vi "StellarNet Init, Read, Close.vi"(0 "Integration Time (ms)":i32=100 caption="Inter scan delay ms", 1 "Use Config\nFile Params (T)":bool, 5 "Number of Scans to Average":i32=1 min=1 max=10000 step=1, 7 "Digitizer Clock Rate Setting":i32=3 min=1 max=3, 9 "Optical Smoothing Level":i32=1 min=0 max=4 step=1, 11 "error in (no error)":errorcluster, 12 "Spectral Channel":i32=1 min=0 max=1 step=1, 14 "Temp  Compensation":bool) -> (4 "Spectrum":cluster{"Wavelengths":dbl[], "buffer out":sgl[]}(graph), 6 "output param":i32, 10 "Critical Error":bool, 15 "error out":errorcluster)   [LabVIEW 2023]
panel:
  # "Use Panel\nParams"
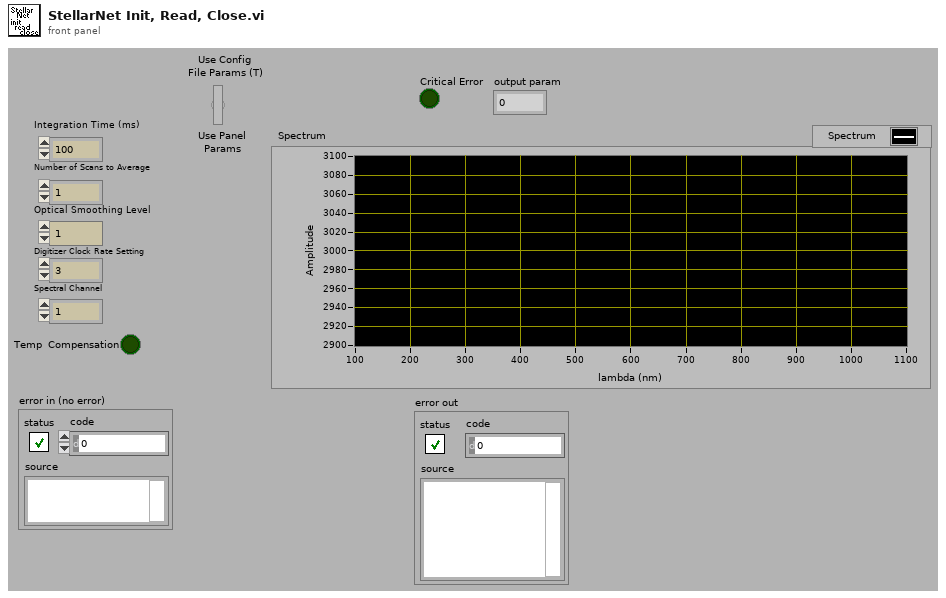
[diagram p1: front panel]
types:
  T1 = cluster{"Coefficients":ext[], "Wavelengths":dbl[]}[]
  T2 = cluster{"Integration Time (ms)":i32, "Number of Scans to Average":i32, "Optical Smoothing Level":i32, "Digitizer Clock Rate Setting":i32, "Temp  Compensation ":bool}[]
  T3 = cluster{"Coefficients":ext[], "Wavelengths":dbl[]}
  T4 = cluster{"Integration Time (ms)":i32, "Number of Scans to Average":i32, "Optical Smoothing Level":i32, "Digitizer Clock Rate Setting":i32, "Temp  Compensation ":bool}
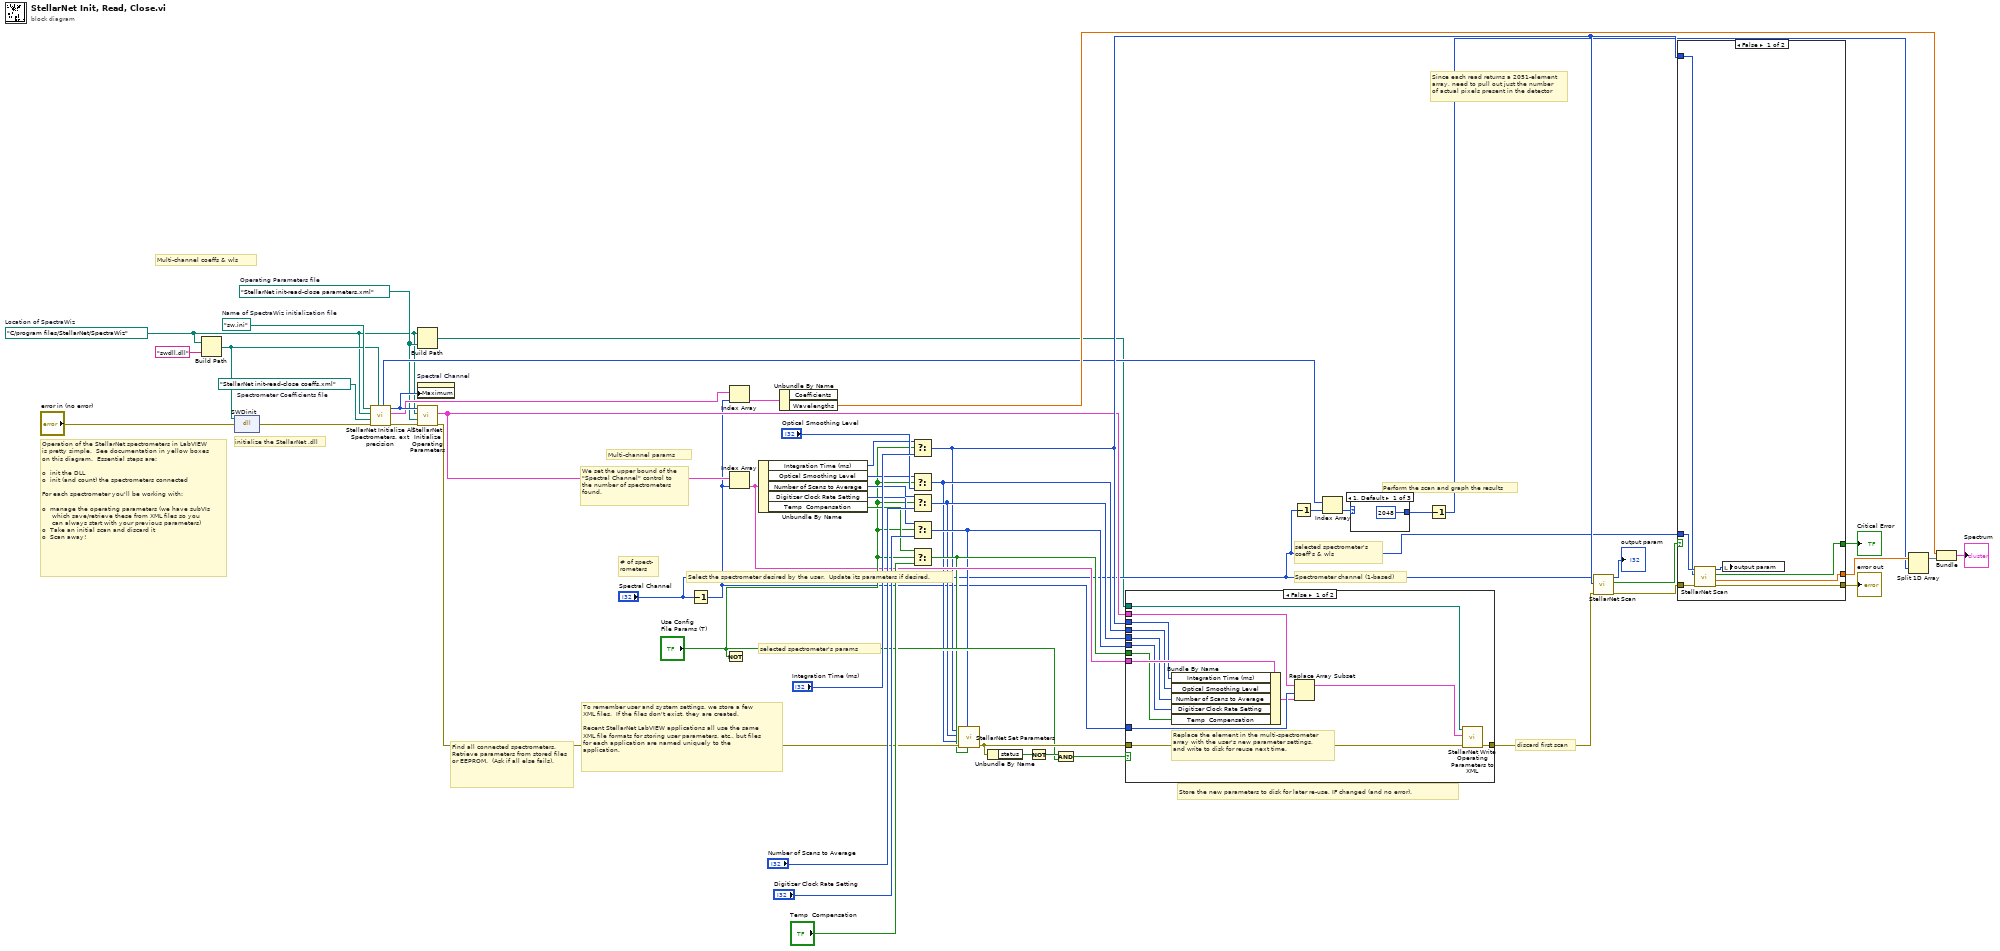
[diagram p0: block diagram]
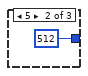
[diagram p2: hidden frame]
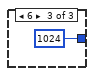
[diagram p3: hidden frame]
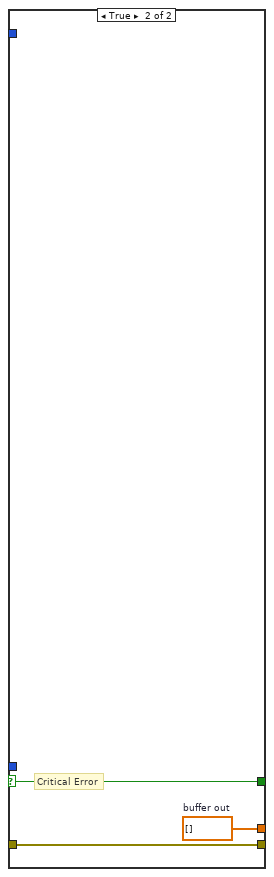
[diagram p5: hidden frame]
diagram:
  w1 = path "C:/program files/StellarNet/SpectraWiz"  # Location of SpectraWiz
  w40 = path "sw.ini"  # Name of SpectraWiz initialization file
  w2 = path "StellarNet init-read-close parameters.xml"  # Operating Parameters file
  w41 = path "StellarNet init-read-close coeffs.xml"  # Spectrometer Coefficients file
  # "Operation of the StellarNet spectrometers in LabVIEW\nis pretty simple.  See documentation in yellow boxes\non this diagram.  Essential steps are:\n\no  init the DLL\no  init (and count) the spectrometers connected\n\nFor each spectrometer you'll be working with:\n\no  manage the operating parameters (we have subVIs\n     which save/retrieve these from XML files so you\n     can always start with your previous parameters)\no  Take an initial scan and discard it\no  Scan away!"
  # "initialize the StellarNet .dll"
  # "Since each read returns a 2051-element\narray, need to pull out just the number\nof actual pixels present in the detector"
  # "Spectrometer channel (1-based)"
  # "Perform the scan and graph the results"
  # "We set the upper bound of the\n\"Spectral Channel\" control to \nthe number of spectrometers \nfound."
  # "To remember user and system settings, we store a few \nXML files.  If the files don't exist, they are created.\n\nRecent StellarNet LabVIEW applications all use the same\nXML file formats for storing user parameters, etc., but files\nfor each application are named uniquely to the \napplication."
  # "Store the new parameters to disk for later re-use, IF changed (and no error)."
  # "Select the spectrometer desired by the user.  Update its parameters if desired."
  # "Find all connected spectrometers.  Retrieve parameters from stored files or EEPROM.  (Ask if all else fails)."
  # "selected spectrometer's\ncoeff's & wls"
  # "Multi-channel coeffs & wls"
  # "selected spectrometer's params"
  # "# of spect-\nrometers"
  # "Multi-channel params"
  # "discard first scan"
  n1 = Build Path(base path=w1, name or relative path="swdll.dll") -> (appended path=w4:path)
  n2 = dll-call lib="C:/Program Files/StellarNet/SpectraWiz/swdll.dll" fn="SWDinit" label="init"(path in=w4, error in="error in (no error)") -> (error out=w6:errorcluster)  [unwired: 2 in, 1 out]
  n3 = call "StellarNet Initialize All Spectrometers, ext precision.vi"("Path of swdll.dll"=w4, "error in"=w6, "Spectrometer Coefficients file"=w41, "Location of SpectraWiz"=w1, "Name of SpectraWiz initialization file"=w40) -> ("error out"=w39:errorcluster, "Multi Channel Coeffs & WLs"=w37:T1, "Number of Channels"=w38:i32, "Detector Types"=w10:u16[])  [unwired: 2 in, 1 out]
  n4 = Build Path(base path=w1, name or relative path=w2) -> (appended path=w3:path)
  n5 = property on="Spectral Channel" class="DigNum (strict)"("Maximum"=w38) -> ()  [unwired: 2 in, 2 out]
  n6 = call "StellarNet Initialize Operating Parameters.vi"("error in"=w39, "Spectrometer Coefficients file"=w2, "Location of SpectraWiz"=w1, "Number of Channels"=w38) -> ("error out"=w35:errorcluster, "Operating Parameters"=w16:T2)  [unwired: 6 in]
  n7 = Decrement(x="Spectral Channel") -> (x-1=w15:i32)
  n8 = Not(x="Use Config\nFile Params (T)") -> ()  [unwired: 1 out]
  n9 = Index Array(array=w37, index=w15) -> (element=w36:T3)
  n10 = Index Array(array=w16, index=w15) -> (element=w22:T4)
  n11 = Unbundle By Name(w22) -> ("Integration Time (ms)"=w33:i32, "Optical Smoothing Level"=w32:i32, "Number of Scans to Average"=w31:i32, "Digitizer Clock Rate Setting"=w30:i32, "Temp  Compensation"=w29:bool)
  n12 = Unbundle By Name(w36) -> ("Wavelengths"=w34:dbl[])  [unwired: 1 out]
  n13 = Select(t=w33, s="Use Config\nFile Params (T)", f="Integration Time (ms)") -> (s? t:f=w17:i32)
  n14 = Select(t=w32, s="Use Config\nFile Params (T)", f="Optical Smoothing Level") -> (s? t:f=w18:i32)
  n15 = Select(t=w31, s="Use Config\nFile Params (T)", f="Number of Scans to Average") -> (s? t:f=w19:i32)
  n16 = Select(t=w30, s="Use Config\nFile Params (T)", f="Digitizer Clock Rate Setting") -> (s? t:f=w20:i32)
  n17 = Select(t=w29, s="Use Config\nFile Params (T)", f="Temp  Compensation") -> (s? t:f=w21:bool)
  n18 = call "StellarNet Set Parameters.vi"("Temp  Compensation"=w21, "Digitizer Clock Rate Setting"=w20, "error in (no error)"=w35, "Optical Smoothing Level"=w18, "Number of Scans to Average"=w19, "Integration Time (ms)"=w17) -> ("error out"=w28:errorcluster)  [unwired: 5 in]
  n19 = Unbundle By Name(w28) -> ("status"=w26:bool)
  n20 = Not(x=w26) -> (.not. x?=w25:bool)
  n21 = And(x=w25, y="Use Config\nFile Params (T)") -> (x .and. y?=w23:bool)
  n22 = case shown="False" w23 {
    tunnel: w28 -> [w55 w67]
    tunnel: [w54 w67] -> w27
    tunnel: w22 -> [w66 _]
    tunnel: w21 -> [w65 _]
    tunnel: w20 -> [w64 _]
    tunnel: w19 -> [w63 _]
    tunnel: w18 -> [w62 _]
    tunnel: w17 -> [w61 _]
    tunnel: w16 -> [w60 _]
    tunnel: w15 -> [w59 _]
    tunnel: w3 -> [w56 _]
    frame False {
      # "Replace the element in the multi-spectrometer\narray with the user's new parameter settings,\nand write to disk for reuse next time."
      n23 = Bundle By Name(cluster=w66, "Integration Time (ms)"=w61, "Optical Smoothing Level"=w62, "Number of Scans to Average"=w63, "Digitizer Clock Rate Setting"=w64, "Temp  Compensation"=w65) -> (w58:T4)
      n24 = Replace Array Subset(array=w60, new element=w58, index=w59) -> (w57:T2)
      n25 = call "StellarNet Write Operating Parameters to XML.vi"("error in (no error)"=w55, "Operating Parameters"=w57, "XML File Path"=w56) -> ("error out"=w54:errorcluster)  [unwired: 8 in]
    }
    frame True {
    }
  }
  n26 = Decrement(x="Spectral Channel") -> (x-1=w12:i32)
  n27 = Index Array(array=w10, index=w12) -> (element=w11:u16)
  n28 = case shown="1, Default" w11 {
    tunnel: [2048 512 1024] -> w8
    frame 1, Default {
    }
    frame 5 {
    }
    frame 6 {
    }
  }
  n29 = Decrement(x=w8) -> (x-1=w7:i32)
  n30 = call "StellarNet Scan.vi"("error in (no error)"=w27, "Integration Time (msec)"=w17, "Spectral Channel"="Spectral Channel") -> ("error out"=w47:errorcluster, "Critical Error"=w48:bool, "output param"=→"output param":i32)  [unwired: 5 in, 1 out]
  n31 = case shown="False" w48 {
    selector: w48 -> [_ w80]
    tunnel: "Spectral Channel" -> [w77 _]
    tunnel: [w76 w79] -> w14
    tunnel: [w74 w80] -> w44
    tunnel: w47 -> [w73 w78]
    tunnel: [w72 w78] -> w46
    tunnel: w17 -> [w71 _]
    frame False {
      n32 = call "StellarNet Scan.vi"("error in (no error)"=w73, "Integration Time (msec)"=w71, "Spectral Channel"=w77) -> ("error out"=w72:errorcluster, "buffer out"=w76:sgl[], "Critical Error"=w74:bool, "output param"=w75:i32)  [unwired: 5 in]
      n33 = local write "output param"(w75) -> ()
    }
    frame True {
      w79 = sgl[] []  # buffer out
      # "Critical Error"
    }
  }
  "error out" <- w46
  "Critical Error" <- w44
  n34 = Split 1D Array(array=w14, index=w7) -> (first subarray=w13:sgl[])  [unwired: 1 out]
  n35 = Bundle("Wavelengths"=w34, w13) -> (→"Spectrum":cluster{"Wavelengths":dbl[], sgl[]})  [unwired: 1 in]
